vi "Check Guest History.vi"(0 "Incoming Rooms Manager Model Interface in":refnum<class "Incoming Rooms Manager Model Interface.lvclass">, 5 "Guest Contact Number In":string caption="Guest Contact Number", 11 "error in (no error)":errorcluster) -> (4 "Incoming Rooms Manager Model Interface out":refnum<class "Incoming Rooms Manager Model Interface.lvclass">, 15 "error out":errorcluster)   [LabVIEW 2023, in "Incoming Rooms Manager Model Interface.lvlib" / "Incoming Rooms Manager Model Interface.lvclass"]
uses:
  Incoming Rooms Manager Model Interface.lvclass
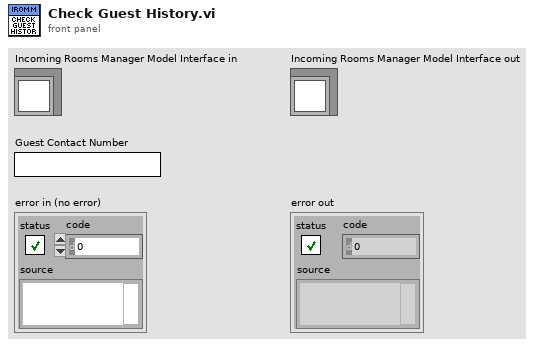
[diagram p1: front panel]
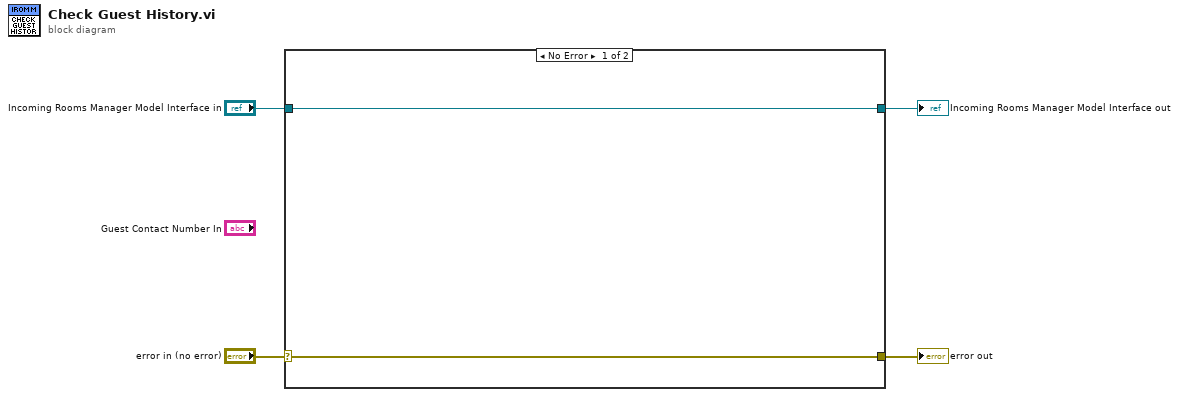
[diagram p0: block diagram]
diagram:
  n1 = case shown="No Error" "error in (no error)" {
    selector: "error in (no error)" -> [w5 w8]
    tunnel: [w5 w8] -> w3
    tunnel: [w6 w7] -> w1
    tunnel: "Incoming Rooms Manager Model Interface in" -> [w6 w7]
    frame No Error {
    }
    frame Error {
    }
  }
  "error out" <- w3
  "Incoming Rooms Manager Model Interface out" <- w1
